vi "FlexRIO1483_8T8.vi"() -> ()   [LabVIEW 2013]
doc: "This is the FPGA VI for the 10-Tap 8-Bit Camera with DRAM example. This example demonstrates how to acquire images from a 10-tap, 8-bit, extended configuration, Camera Link camera and transfer the images to the host. This example supports area scan and line scan cameras for both continuous and finite acquisitions.\n\nThis example also demonstrates the use of DRAM as a frame buffer for very high speed acquisitions. Data packing and flow-control are also employed to maximize use of the available DRAM and FIFOs in terms of both memory space and performance.\n\nAdditionally, the example demonstrates the serial server, which allows third-party camera configuration utilities to communicate with the camera using the Camera Link serial interface while this VI is running."
uses:
  <vilib>/Platform/TimedLoop/XDataNode/timing_clust.ctl
  <vilib>/Platform/TimedLoop/XDataNode/nitl_modes.ctl
  <vilib>/Platform/TimedLoop/XDataNode/wakeup.ctl
  <vilib>/rvi/eio/common/nirviEmuTemplateMethod_errors.vi
  <vilib>/rvi/Emulation/niFpgaSctlEmulationGetInTimedLoop.vi
  <vilib>/rvi/Emulation/niFpgaEmulationReportErrorSimple.vi
  <vilib>/rvi/Emulation/niFpgaGetClockAttributes.vi
  <vilib>/rvi/Emulation/niFpgaCriticalErrorInLSC.vi
  Common/CL Data to Pixels/8 Tap 8-Bit.vi
  <vilib>/rvi/interface/RandomDataEmulation/nirviRandomDataFPGAFIFO.vi
  <vilib>/rvi/interface/RandomDataEmulation/niFpgaRandomDataHandleErrors.vi
  <vilib>/rvi/Emulation/niFpgaProcessEmulError.vi
  <vilib>/Platform/TimedLoop/XDataNode/XDataNode.xnode
  <vilib>/eio/EIONode/EIONode.xnode
  <vilib>/rvi/DataTransferAndStorage/Container/XNode/niFpgaContainer.xnode
  <vilib>/rvi/interface/RandomDataEmulation/nirviRandomDataFpgaReadWriteTemplate.vi
  <vilib>/Platform/TimedLoop/XDataNode/XDNodeRunTimeDep.lvlib
panel:
  in  "Tab Control":T1(tab)
  out "Platform":enum8{"FlexRIO", "cRIO", "RSeries"}(ring)
  out "FPGAVIversion":u8[](array[numeric])=[1, 1]
  out "InitDone":bool
  out "InsertedIOModule ID":u32=278099145
  out "RIOAdapterCorrect":bool
  out "Fref":u32=100000000
  out "DevTemp":i16=147
  out "DevProfile":u8=1
  in  "DAQStartStop":bool
  in  "DebugMode":bool
  out "DevQualityStatus":u8
  out "DMATtoHOSTNCh":u16[](array[numeric])=[1]
  in  "DMATtoHOSTEnable0":bool
  out "DMATtoHOSTOverflows":u16
  out "DMATtoHOSTFrameType":u8[](array[numeric])
  out "DMATtoHOSTSampleSize":u8[](array[numeric])=[1]
  in  "SpareHigh":bool=TRUE caption="CL Config.Spare Active High"
  in  "FVALHigh":bool=TRUE caption="CL Config.FVAL Active High"
  in  "LVALHigh":bool=TRUE caption="CL Config.LVAL Active High"
  in  "DVALHigh":bool=TRUE caption="CL Config.DVAL Active High"
  in  "LineScan":bool caption="CL Config.Line Scan"
  in  "SignalMapping":u8 caption="CL Config.Signal Mapping"
  in  "Configuration":u8=2 caption="CL Config.Configuration"
  in  "ControlEnable":bool=TRUE caption="IO Module\\CL Control Enable"
  in  "uartReceive":bool caption="UART.Receive"
  out "uartRxByte":u8 caption="UART.Rx Data" format="%02x"
  out "uartTxReady":bool caption="UART.Tx Ready"
  out "uartOverrunError":bool caption="UART.Overrun Error"
  out "uartFramingError":bool caption="UART.Framing Error"
  out "uartBreakIndicator":bool caption="UART.Break Indicator"
  out "uartRxReady":bool caption="auxDI1"
  in  "uartByteMode":bool=TRUE caption="UART.Byte Mode"
  in  "uartSetBaudRate":bool caption="UART.Set Baud Rate"
  in  "uartTransmit":bool caption="UART.Transmit"
  in  "uartBaudRate":u8=1 caption="UART.Baud Rate"
  in  "uartTxByte":u8=1 caption="DataBytetoTx" format="%x"
  out "DI0":bool
  out "DI1":bool
  in  "auxAO0":i16
  out "auxAI1":i16
  out "SGNo":u8
  in  "DO0":bool
  in  "DO1":bool
  out "auxAI0":i16
  out "Acq Status.Lines Per Frame":u32
  out "Acq Status.Frames Acq'd":u32
  out "Acq Status.Clocks Per Line":u32
  out "Acq Status.Acq In Progress":bool
  in  "Acq Control.Ignore DVAL":bool
  in  "Acq Control.Frames To Acq":u32
  in  "Acq Control.Line Scan Height":u32
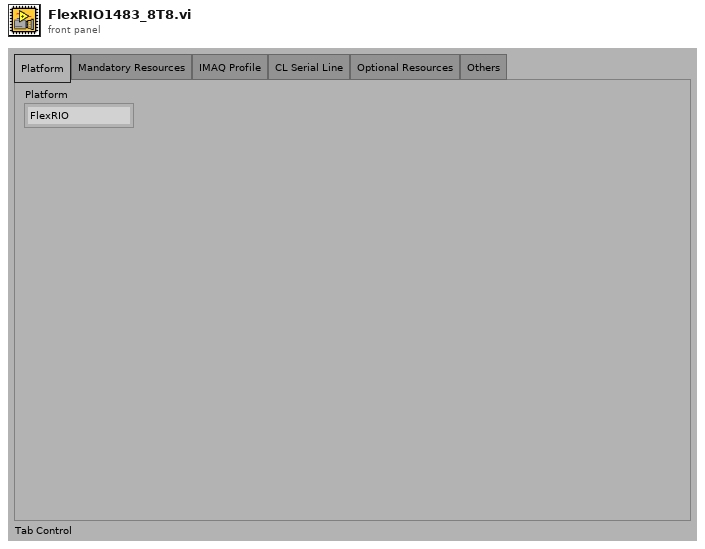
[diagram p1: front panel]
types:
  T1 = enum32{"Platform", "Mandatory Resources", "IMAQ Profile", "CL Serial Line", "Optional Resources", "Others"}
  T2 = typedef "XDNodeRunTimeDep.lvlib/timing_clust.ctl" = cluster{"Expected End [f-1]":u64, "Actual End [f-1]":u64, "Finished Late? [f-1]":bool, "Expected End [i-1]":u64, "Actual End [i-1]":u64, "Finished Late? [i-1]":bool, "Expected Start [i]":u64, "Actual Start [i]":u64, "Expected Start [f]":u64, "Actual Start [f]":u64, "Source Name":string, "Structure Name":string, "Period":i64, "Deadline":i64, "Offset":i64, "Start":i64, "Priority":i32, "Timeout":i32, "Mode":T3, "Wakeup Reason":T4, "Error":errorcluster, "Source Type":string, "Secondary Source Type":string, "Global End Time":u64, "Global Start Time":u64, "Frame Duration":u64, "Iteration Duration":u64, "Assigned CPU":i32, "I/O Scan Engine Mode":u32}
  T3 = typedef "XDNodeRunTimeDep.lvlib/nitl_modes.ctl" = enum32{"No Change", "Process missed periods, maintain original phase", "Discard missed periods, maintain original phase", "Process missed periods, ignore original phase", "Discard missed periods, ignore original phase"}
  T4 = typedef "XDNodeRunTimeDep.lvlib/wakeup.ctl" = enum32{"Normal", "Aborted", "Asynchronous wakeup", "Timing source error", "Timed loop error", "Timeout"}
  T5 = cluster{"Enables Valid":bool, "Frame Valid":bool, "Line Valid":bool, "Data Valid":bool}
  T6 = enum8{"Standard", "Basler 10-tap", "Vosskühler 10-tap"}
  T7 = cluster{"Pixel 0":u8, "Pixel 1":u8, "Pixel 2":u8, "Pixel 3":u8, "Pixel 4":u8, "Pixel 5":u8, "Pixel 6":u8, "Pixel 7":u8}
  T8 = cluster{"Tx Data":u8[], "Transmit":bool, "Receive":bool, "Byte Mode":bool, "Set Baud Rate":bool, "Baud Rate":u8}
  T9 = cluster{"Rx Data":u8, "Turn Off Transmit":bool, "Turn Off Receive":bool, "Turn Off Set Baud Rate":bool, "Tx Ready":bool, "Rx Ready":bool, "Break Indicator":bool, "Framing Error":bool, "Overrun Error":bool}
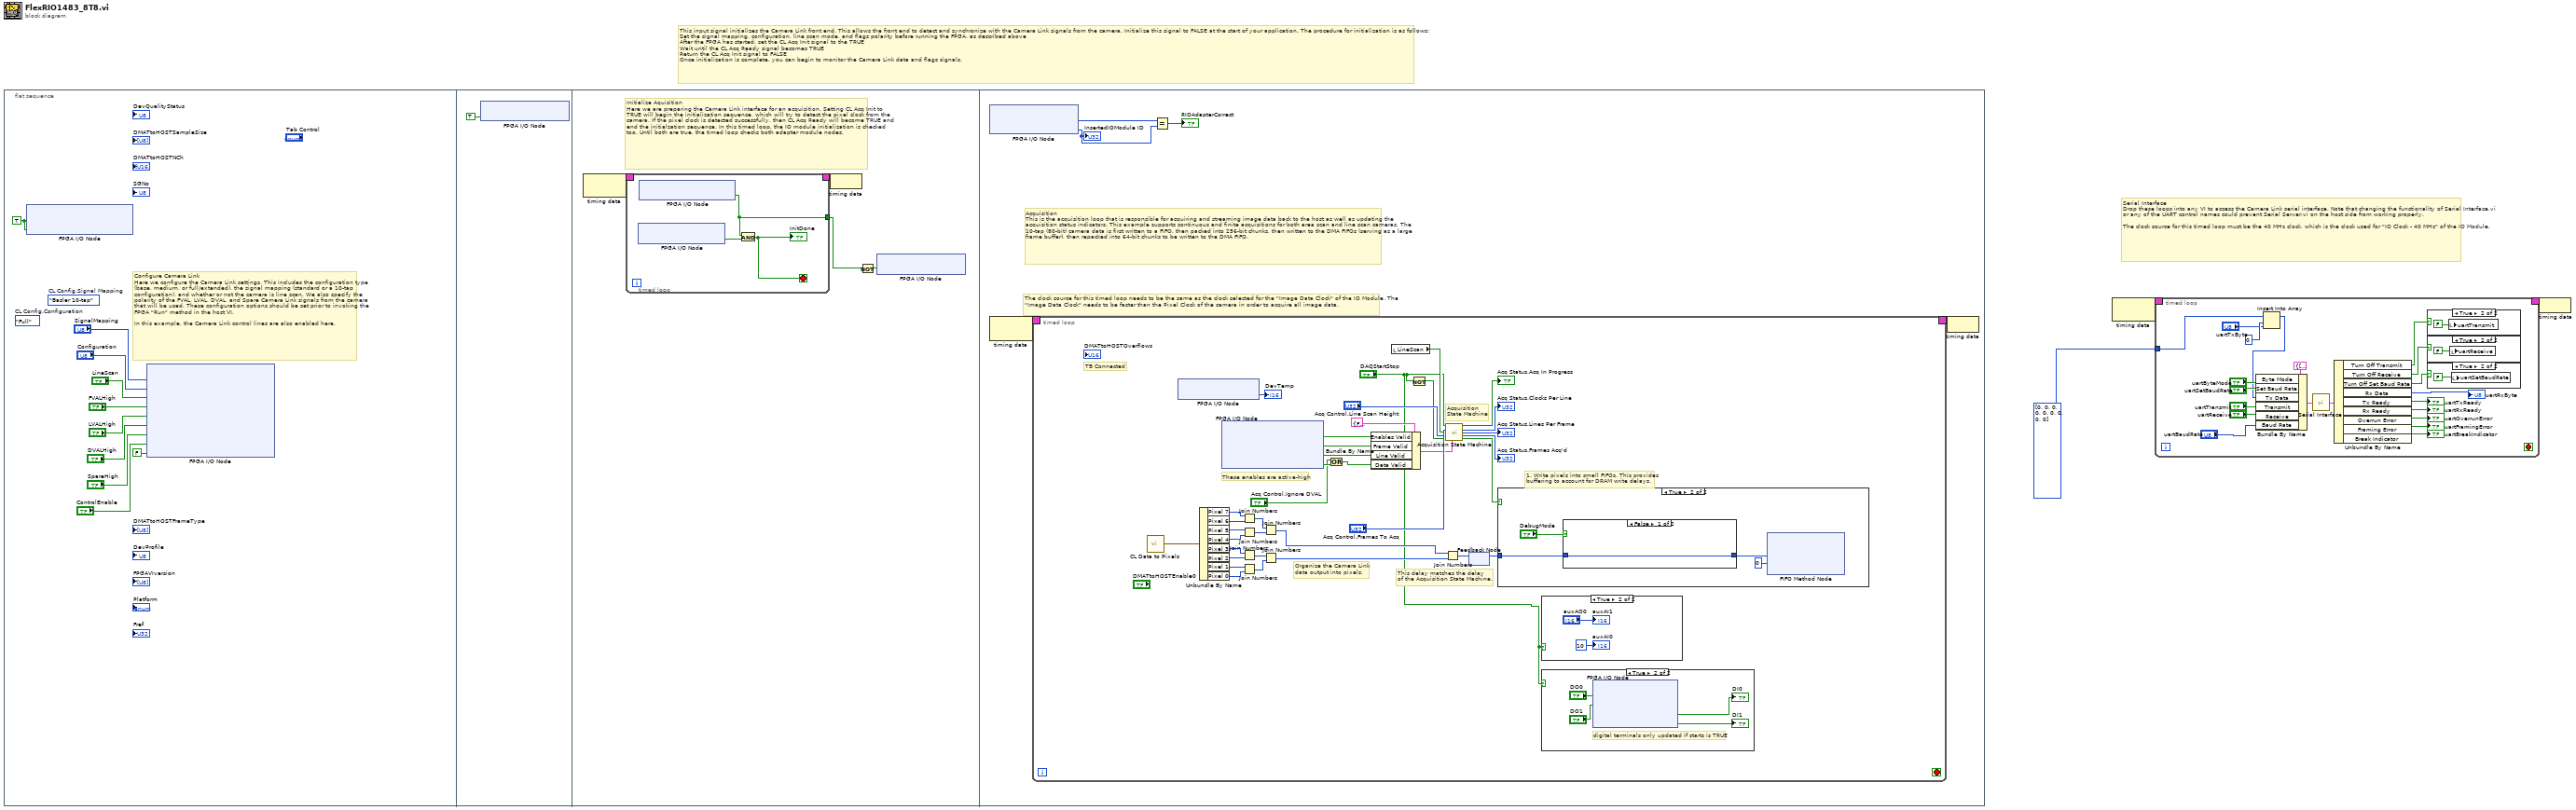
[diagram p0: block diagram]
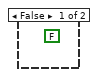
[diagram p7: hidden frame]
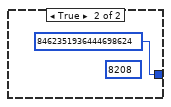
[diagram p8: hidden frame]
diagram:
  # "This input signal initializes the Camera Link front end. This allows the front end to detect and synchronize with the Camera Link signals from the camera. Initialize this signal to FALSE at the start of your application. The procedure for initialization is as follows: \nSet the signal mapping, configuration, line scan mode, and flags polarity before running the FPGA, as described above \nAfter the FPGA has started, set the CL Acq Init signal to the TRUE \nWait until the CL Acq Ready signal becomes TRUE \nReturn the CL Acq Init signal to FALSE \nOnce initialization is complete, you can begin to monitor the Camera Link data and flags signals."
  # "Serial Interface\nDrop these loops into any VI to access the Camera Link serial interface. Note that changing the functionality of Serial Interface.vi or any of the UART control names could prevent Serial Server.vi on the host side from working properly.\n\nThe clock source for this timed loop must be the 40 MHz clock, which is the clock used for \"IO Clock - 40 MHz\" of the IO Module."
  n1 = flat-sequence {
    frame #0 {
      w4 = TRUE ("IO Module\\TTL Out Enable 0")
      (unwired) T6."Basler 10-tap"  # CL Config.Signal Mapping
      (unwired) enum8{"Base", "Medium", "Full"}."Full"  # CL Config.Configuration
      # "Configure Camera Link\nHere we configure the Camera Link settings. This includes the configuration type (base, medium, or full/extended), the signal mapping (standard or a 10-tap configuration), and whether or not the camera is line scan. We also specify the polarity of the FVAL, LVAL, DVAL, and Spare Camera Link signals from the camera that will be used. These configuration options should be set prior to invoking the FPGA \"Run\" method in the host VI.\n\nIn this example, the Camera Link control lines are also enabled here."
      n2 = xnode "FPGA I/O Node"("IO Module\\TTL Out Enable 0"=w4, "IO Module\\TTL Out Enable 1"=w4) -> ()  [unwired: 2 in, 2 out]
      n3 = xnode "FPGA I/O Node"("IO Module\\CL Set Signal Mapping"="SignalMapping", "IO Module\\CL Set Configuration"="Configuration", "IO Module\\CL Set Line Scan"="LineScan", "IO Module\\CL Set FVAL Active High"="FVALHigh", "IO Module\\CL Set LVAL Active High"="LVALHigh", "IO Module\\CL Set DVAL Active High"="DVALHigh", "IO Module\\CL Set Spare Active High"="SpareHigh", "IO Module\\CL Control Enable"="ControlEnable", "IO Module\\CL Acq Init"=FALSE ("IO Module\\CL Acq Init")) -> ()  [unwired: 9 in, 9 out]
    }
    frame #1 {
      n4 = xnode "FPGA I/O Node"("IO Module\\CL Acq Init"=TRUE) -> ()  [unwired: 1 in, 1 out]
    }
    frame #2 {
      # "Initialize Aquisition\nHere we are preparing the Camera Link interface for an acquisition. Setting CL Acq Init to TRUE will begin the initialization sequence, which will try to detect the pixel clock from the camera. If the pixel clock is detected successfully, then CL Acq Ready will become TRUE and end the initialzation sequence. In this timed loop, the IO module initialization is checked too. Until both are true, the timed loop checks both adapter module nodes."
      n5 = node-c288() -> (w18:T2)  [unwired: 1 out]
      n6 = timed-loop {
        timing: w18 -> [_]
        timing-out: [_] -> w17
        tunnel: [w19] -> w15
        stop <- w21 stop-if-true
        n7 = xnode "FPGA I/O Node"() -> ("IO Module IO Enabled"=w20:bool)  [unwired: 1 in, 1 out]
        n8 = xnode "FPGA I/O Node"() -> ("IO Module\\CL Acq Ready"=w19:bool)  [unwired: 1 in, 1 out]
        n9 = And(x=w19, y=w20) -> (x .and. y?=w21:bool)
        "InitDone" <- w21
      }
      n10 = node-c288(w17) -> ()
      n11 = Not(x=w15) -> (.not. x?=w16:bool)
      n12 = xnode "FPGA I/O Node"("IO Module\\CL Acq Init"=w16) -> ()  [unwired: 1 in, 1 out]
    }
    frame #3 {
      # "The clock source for this timed loop needs to be the same as the clock selected for the \"Image Data Clock\" of the IO Module. The \"Image Data Clock\" needs to be faster than the Pixel Clock of the camera in order to acquire all image data."
      # "Acquisition\nThis is the acquisition loop that is responsible for acquiring and streaming image data back to the host as well as updating the acquisition status indicators. This example supports continuous and finite acquisitions for both area scan and line scan cameras. The 10-tap (80-bit) camera data is first written to a FIFO, then packed into 256-bit chunks, then written to the DMA FIFOs (serving as a large frame buffer), then repacked into 64-bit chunks to be written to the DMA FIFO."
      n13 = xnode "FPGA I/O Node"() -> ("Expected IO Module ID"=w28:u32, "Inserted IO Module ID"=w27:u32)  [unwired: 2 in, 2 out]
      "InsertedIOModule ID" <- w27
      n14 = node-c288() -> (w30:T2)  [unwired: 1 in]
      n15 = timed-loop {
        timing: w30 -> [_]
        timing-out: [_] -> w29
        stop <- _ stop-if-true
        # "TB Connected"
        # "1. Write pixels into small FIFOs. This provides\nbuffering to account for DRAM write delays."
        # "Organize the Camera Link\ndata output into pixels."
        # "These enables are active-high"
        # "This delay matches the delay\nof the Acquisition State Machine."
        # "Acquisition\nState Machine"
        n16 = call-poly "CL Data to Pixels.vi"() -> ("Pixels"=w66:T7)  [unwired: 1 in]
        n17 = xnode "FPGA I/O Node"() -> ("Device Temperature"=→"DevTemp":i16)  [unwired: 1 in, 1 out]
        n18 = Unbundle By Name(w66) -> ("Pixel 7"=w48:u8, "Pixel 6"=w47:u8, "Pixel 5"=w46:u8, "Pixel 4"=w45:u8, "Pixel 3"=w44:u8, "Pixel 2"=w43:u8, "Pixel 1"=w42:u8, "Pixel 0"=w41:u8)
        n19 = xnode "FPGA I/O Node"() -> ("IO Module\\CL Output Valid"=w58:bool, "IO Module\\CL Frame Valid"=w57:bool, "IO Module\\CL Line Valid"=w56:bool, "IO Module\\CL Data Valid"=w53:bool)  [unwired: 4 in, 4 out]
        n20 = Join Numbers(hi=w48, lo=w47) -> ((hi.lo)=w39:u16)
        n21 = Join Numbers(hi=w46, lo=w45) -> ((hi.lo)=w38:u16)
        n22 = Join Numbers(hi=w44, lo=w43) -> ((hi.lo)=w37:u16)
        n23 = Join Numbers(hi=w42, lo=w41) -> ((hi.lo)=w40:u16)
        n24 = Join Numbers(hi=w39, lo=w38) -> ((hi.lo)=w36:u32)
        n25 = Join Numbers(hi=w37, lo=w40) -> ((hi.lo)=w35:u32)
        n26 = Or(x="Acq Control.Ignore DVAL", y=w53) -> (x .or. y?=w52:bool)
        n27 = Bundle By Name(cluster=T5 {"Enables Valid"=FALSE, "Frame Valid"=FALSE, "Line Valid"=FALSE, "Data Valid"=FALSE} ("Enables"), "Enables Valid"=w58, "Frame Valid"=w57, "Line Valid"=w56, "Data Valid"=w52) -> (w55:T5)
        n28 = local read "LineScan"() -> (w50:bool)
        n29 = Not(x="DAQStartStop") -> (.not. x?=w33:bool)
        n30 = Join Numbers(hi=w36, lo=w35) -> ((hi.lo)=w34:u64)
        n31 = call "Acquisition State Machine.vi"("Acquire"="DAQStartStop", "Frames to Acquire"="Acq Control.Frames To Acq", "Line Scan"=w50, "Line Scan Height"="Acq Control.Line Scan Height", "Cancel Acq"=w33, "Enables"=w55) -> ("Acq In Progress"=→"Acq Status.Acq In Progress":bool, "Num Clocks Per Line"=→"Acq Status.Clocks Per Line":u32, "Num Lines Per Frame"=→"Acq Status.Lines Per Frame":u32, "Num Frames Acq'd"=→"Acq Status.Frames Acq'd":u32, "Capture Cycle"=w64:bool)  [unwired: 4 in, 1 out]
        n32 = feedback-in #1(w34) -> ()
        n33 = feedback #1() -> (w65:u64)  [unwired: 1 in]
        n34 = case shown="True" w64 {
          tunnel: w65 -> [_ w74]
          frame False {
            (unwired) FALSE ("Timed Out?")
          }
          frame True {
            n35 = case shown="False" "DebugMode" {
              tunnel: w74 -> [w77 _]
              tunnel: [w77 u64 8462351936444698624] -> w73
              frame False {
              }
              frame True {
                (unwired) u16 8208
              }
            }
            n36 = xnode ("FIFO Method Node")("Element"=w73, "Timeout"=0) -> ()  [unwired: 1 in, 2 out]
          }
        }
        n37 = case shown="True" "DAQStartStop" {
          frame False {
          }
          frame True {
            "auxAI0" <- i16 10 ("auxAI0")
            "auxAI1" <- "auxAO0"
          }
        }
        n38 = case shown="True" "DAQStartStop" {
          frame False {
          }
          frame True {
            # "digital terminals only updated if starts is TRUE"
            n39 = xnode "FPGA I/O Node"("IO Module\\TTL Out 0"="DO0", "IO Module\\TTL Out 1"="DO1") -> ("IO Module\\TTL In 2"=→"DI0":bool, "IO Module\\TTL In 3"=→"DI1":bool)  [unwired: 4 in, 4 out]
          }
        }
      }
      n40 = Equal?(x=w28, y=w27) -> (x = y?=→"RIOAdapterCorrect":bool)
      n41 = node-c288(w29) -> ()
    }
  }
  n42 = node-c288() -> (w3:T2)  [unwired: 1 out]
  n43 = timed-loop {
    timing: w3 -> [_]
    timing-out: [_] -> w2
    tunnel: u8[] [0, 0, 0, 0, 0, 0, 0, 0, 0] -> [w87]
    stop <- _ stop-if-true
    n44 = Insert Into Array(array=w87, index=0, new element="uartTxByte") -> (w86:u8[])
    n45 = Bundle By Name(cluster=T8 {"Tx Data"=[0, 0, 0, 0, 0, 0, 0, 0, 0, 0], "Transmit"=FALSE, "Receive"=FALSE, "Byte Mode"=TRUE, "Set Baud Rate"=FALSE, "Baud Rate"=0} ("UART Inputs"), "Byte Mode"="uartByteMode", "Set Baud Rate"="uartSetBaudRate", "Tx Data"=w86, "Transmit"="uartTransmit", "Receive"="uartReceive", "Baud Rate"="uartBaudRate") -> (w89:T8)
    n46 = call "Serial Interface.vi"("UART Inputs"=w89) -> ("UART Outputs"=w99:T9)
    n47 = Unbundle By Name(w99) -> ("Turn Off Transmit"=w92:bool, "Turn Off Receive"=w93:bool, "Turn Off Set Baud Rate"=w91:bool, "Rx Data"=→"uartRxByte":u8, "Tx Ready"=→"uartTxReady":bool, "Rx Ready"=→"uartRxReady":bool, "Overrun Error"=→"uartOverrunError":bool, "Framing Error"=→"uartFramingError":bool, "Break Indicator"=→"uartBreakIndicator":bool)
    n48 = case shown="True" w92 {
      frame False {
      }
      frame True {
        n49 = local write "uartTransmit"(FALSE ("UART.Transmit")) -> ()
      }
    }
    n50 = case shown="True" w93 {
      frame False {
      }
      frame True {
        n51 = local write "uartReceive"(FALSE ("UART.Receive")) -> ()
      }
    }
    n52 = case shown="True" w91 {
      frame False {
      }
      frame True {
        n53 = local write "uartSetBaudRate"(FALSE ("UART.Receive")) -> ()
      }
    }
  }
  n54 = node-c288(w2) -> ()
